vi "Sample Pad Example (LINX).vi"() -> ()   [LabVIEW 2020]
doc: "A simple sample pad, which can trigger up to 16 simultaneous sound effects. Demonstrates the Mixer component, including file loading, playback, and mixer audio monitoring via a music visualizer."
uses:
  Mixer/Channel/Controls/Channel State.ctl
  Mixer/Mixer/Mixer.lvclass/Mixer.ctl
  <vilib>/MakerHub/LINX/Public/Peripherals/Digital/Digital Read N Chans.vi
  e8fa8eb6-c38c-4b8a-b362-922d187964a0.vi
  <vilib>/MakerHub/LINX/Private/Local IO/LinxDigitalRead.vi
  <vilib>/MakerHub/LINX/Public/Utilities/Check Channel.vi
  Mixer/Mixer/Polymorphic VIs/Channel Load (Path).vi
  <vilib>/MakerHub/LINX/Public/Utilities/Open Local.vi
  <vilib>/MakerHub/LINX/Private/Utilties/Generate Error.vi
  Mixer/Mixer/Mixer.lvclass
  Mixer/Channel/Channel.lvclass
  <vilib>/MakerHub/LINX/LMH-LINX.lvlib
panel:
  in  "Sample Path":path=path "/home/pi/samples"
  in  "Stop":bool
  in  "Play 4":bool caption="V"
  in  "Play 3":bool caption="C"
  in  "Play 2":bool caption="X"
  in  "Play 1":bool caption="Z"
  in  "Play 8":bool caption="F"
  in  "Play 7":bool caption="D"
  in  "Play 6":bool caption="S"
  in  "Play 5":bool caption="A"
  in  "Play 12":bool caption="R"
  in  "Play 11":bool caption="E"
  in  "Play 10":bool caption="W"
  in  "Play 9":bool caption="Q"
  in  "Play 16":bool caption="4"
  in  "Play 15":bool caption="3"
  in  "Play 14":bool caption="2"
  in  "Play 13":bool caption="1"
  # "Instructions:\n1. Ensure G-Audio has been installed on the LINX target.\n2. Enter the path to a folder of audio files on the LINX target\n    (e.g. /home/pi/samples).\n3. Run the VI.\n4. Click the buttons below to trigger playback.\n5. (Optional) Wire buttons to the device's DI channels."
  # "G"
  # "-Audio"
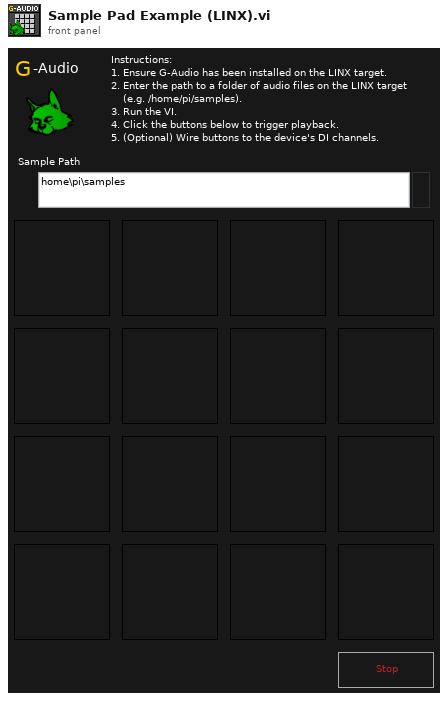
[diagram p1: front panel]
types:
  T1 = typedef "G-Audio.lvlib/Channel.lvclass/Channel State.ctl" = enum16{"Empty", "Error", "Loading", "Loaded", "Stopped", "Paused", "Playing", "Retrigger"}
  T2 = typedef "LMH-LINX.lvlib/LINX Ref.ctl" = cluster{"IO":T3, "Interface":T4, "LINX Device Config":T5}
  T3 = typedef "LMH-LINX.lvlib/Platform.ctl" = enum16{"Remote", "Local"}
  T4 = typedef "LMH-LINX.lvlib/Interface.ctl" = enum16{"Serial", "TCP"}
  T5 = typedef "LMH-LINX.lvlib/Device.lvlib/LINX Device Config.ctl" = cluster{"Interface":T4, "COM Port":refnum<visa-resource-name>, "TCP Configuration":T6, "Device Family":u8, "Device ID":u8, "Device Name":string, "TCP Ref":refnum<k5>, "Channels":T7}
  T6 = typedef "LMH-LINX.lvlib/Device.lvlib/TCP Config.ctl" = cluster{"IP Address":string, "Port":u16}
  T7 = typedef "LMH-LINX.lvlib/Channels.ctl" = cluster{"DI":u8[], "DO":u8[], "AI":u8[], "AO":u8[], "PWM":u8[], "QE":u8[], "UART":u8[], "I2C 2":u8[], "SPI":u8[], "CAN":u8[], "Servo":u8[], "AI Ref (V)":dbl, "AI Resolution (Bits)":u8, "AO Ref (V)":dbl, "AO Resolution (Bits)":u8}
  T8 = typedef "G-Audio.lvlib/Channel.lvclass/Channel Status.ctl" = cluster{"Frame":u64, "State":T1, "Volume":dbl}
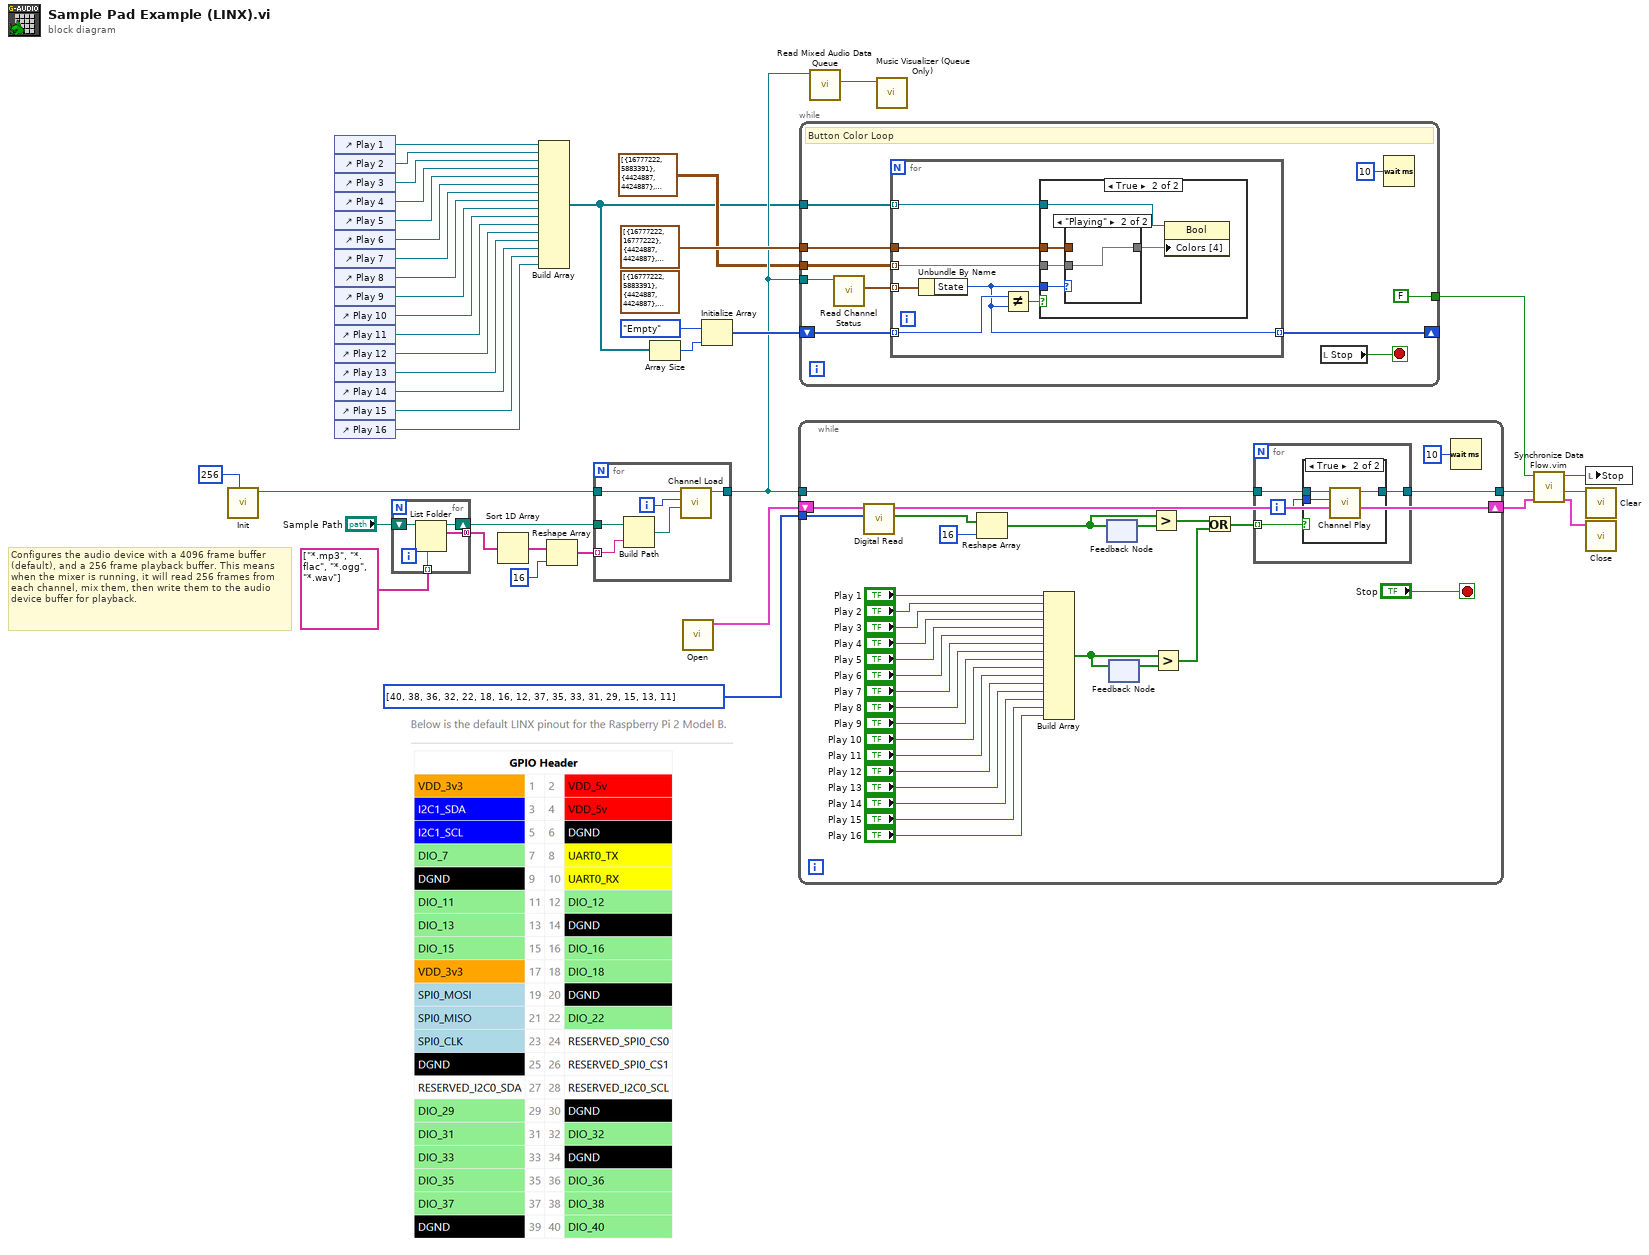
[diagram p0: block diagram]
diagram:
  (unwired) cluster{"Color Box":u32, "Color Box":u32}[][] [[{"Color Box"=16777222, "Color Box"=5883391}, {"Color Box"=4424887, "Color Box"=4424887}, {"Color Box"=4424887, "Color Box"=4424887}, {"Color Box"=4424887, "Color Box"=4424887}], [{"Color Box"=16777222, "Color Box"=5883391}, {"Color Box"=4424887, "Color Box"=4424887}, {"Color Box"=4424887, "Color Box"=4424887}, {"Color Box"=4424887, "Color Box"=4424887}], [{"Color Box"=16777222, "Color Box"=5883391}, {"Color Box"=4424887, "Color Box"=4424887}, {"Color Box"=4424887, "Color Box"=4424887}, {"Color Box"=4424887, "Color Box"=4424887}], [{"Color Box"=16777222, "Color Box"=5883391}, {"Color Box"=4424887, "Color Box"=4424887}, {"Color Box"=4424887, "Color Box"=4424887}, {"Color Box"=4424887, "Color Box"=4424887}], [{"Color Box"=16777222, "Color Box"=6618880}, {"Color Box"=4424887, "Color Box"=4424887}, {"Color Box"=4424887, "Color Box"=4424887}, {"Color Box"=4424887, "Color Box"=4424887}], [{"Color Box"=16777222, "Color Box"=6618880}, {"Color Box"=4424887, "Color Box"=4424887}, {"Color Box"=4424887, "Color Box"=4424887}, {"Color Box"=4424887, "Color Box"=4424887}], [{"Color Box"=16777222, "Color Box"=6618880}, {"Color Box"=4424887, "Color Box"=4424887}, {"Color Box"=4424887, "Color Box"=4424887}, {"Color Box"=4424887, "Color Box"=4424887}], [{"Color Box"=16777222, "Color Box"=6618880}, {"Color Box"=4424887, "Color Box"=4424887}, {"Color Box"=4424887, "Color Box"=4424887}, {"Color Box"=4424887, "Color Box"=4424887}], [{"Color Box"=16777222, "Color Box"=16746514}, {"Color Box"=4424887, "Color Box"=4424887}, {"Color Box"=4424887, "Color Box"=4424887}, {"Color Box"=4424887, "Color Box"=4424887}], [{"Color Box"=16777222, "Color Box"=16746514}, {"Color Box"=4424887, "Color Box"=4424887}, {"Color Box"=4424887, "Color Box"=4424887}, {"Color Box"=4424887, "Color Box"=4424887}], [{"Color Box"=16777222, "Color Box"=16746514}, {"Color Box"=4424887, "Color Box"=4424887}, {"Color Box"=4424887, "Color Box"=4424887}, {"Color Box"=4424887, "Color Box"=4424887}], [{"Color Box"=16777222, "Color Box"=16746514}, {"Color Box"=4424887, "Color Box"=4424887}, {"Color Box"=4424887, "Color Box"=4424887}, {"Color Box"=4424887, "Color Box"=4424887}], [{"Color Box"=16777222, "Color Box"=16711680}, {"Color Box"=4424887, "Color Box"=4424887}, {"Color Box"=4424887, "Color Box"=4424887}, {"Color Box"=4424887, "Color Box"=4424887}], [{"Color Box"=16777222, "Color Box"=16711680}, {"Color Box"=4424887, "Color Box"=4424887}, {"Color Box"=4424887, "Color Box"=4424887}, {"Color Box"=4424887, "Color Box"=4424887}], [{"Color Box"=16777222, "Color Box"=16711680}, {"Color Box"=4424887, "Color Box"=4424887}, {"Color Box"=4424887, "Color Box"=4424887}, {"Color Box"=4424887, "Color Box"=4424887}], [{"Color Box"=16777222, "Color Box"=16711680}, {"Color Box"=4424887, "Color Box"=4424887}, {"Color Box"=4424887, "Color Box"=4424887}, {"Color Box"=4424887, "Color Box"=4424887}]] ("appended array")
  # "Configures the audio device with a 4096 frame buffer (default), and a 256 frame playback buffer. This means when the mixer is running, it will read 256 frames from each channel, mix them, then write them to the audio device buffer for playback."
  n1 = call "Init.vi"("Playback Size (4096)"=256) -> ("Mixer out"=w6:refnum<class "Mixer.lvclass">)  [unwired: 9 in, 1 out]
  n2 = control-ref of="Play 1"() -> (w30:refnum<vi>)
  n3 = control-ref of="Play 2"() -> (w29:refnum<vi>)
  n4 = control-ref of="Play 3"() -> (w28:refnum<vi>)
  n5 = control-ref of="Play 4"() -> (w27:refnum<vi>)
  n6 = control-ref of="Play 5"() -> (w26:refnum<vi>)
  n7 = control-ref of="Play 6"() -> (w25:refnum<vi>)
  n8 = control-ref of="Play 7"() -> (w24:refnum<vi>)
  n9 = control-ref of="Play 8"() -> (w23:refnum<vi>)
  n10 = control-ref of="Play 9"() -> (w22:refnum<vi>)
  n11 = control-ref of="Play 10"() -> (w21:refnum<vi>)
  n12 = control-ref of="Play 11"() -> (w20:refnum<vi>)
  n13 = control-ref of="Play 12"() -> (w19:refnum<vi>)
  n14 = control-ref of="Play 13"() -> (w18:refnum<vi>)
  n15 = control-ref of="Play 14"() -> (w17:refnum<vi>)
  n16 = control-ref of="Play 15"() -> (w16:refnum<vi>)
  n17 = control-ref of="Play 16"() -> (w15:refnum<vi>)
  n18 = for {
    shift-right: [w45] -> w11
    shift-left: "Sample Path" -> [w44]
    tunnel: string[] ["*.mp3", "*.flac", "*.ogg", "*.wav"] -> [w43] mode=indexing
    tunnel: [w42] -> w8 mode=concatenating
    n19 = List Folder(path=w44, pattern=w43) -> (path out=w45:path, filenames=w42:string[])  [unwired: 2 in, 2 out]
  }
  n20 = Sort 1D Array(array=w8) -> (sorted array=w7:string[])
  n21 = Build Array(w30, w29, w28, w27, w26, w25, w24, w23, w22, w21, w20, w19, w18, w17, w16, w15) -> (w1:refnum<vi>[])
  n22 = Reshape Array(w7, 16 ("dimension size")) -> (w12:string[])
  n23 = for {
    tunnel: w12 -> [w51] mode=indexing
    tunnel: w11 -> [w50]
    tunnel: w6 -> [w49]
    tunnel: [w46] -> w4
    i -> [w48]
    n24 = Build Path(base path=w50, name or relative path=w51) -> (appended path=w47:path)
    n25 = call-poly "Channel Load.vi"("Path"=w47, "Channel Index"=w48, "Mixer in"=w49) -> ("Mixer out"=w46:refnum<class "Mixer.lvclass">)  [unwired: 7 in, 1 out]
  }
  n26 = Array Size(array=w1) -> (size(s)=w36:i32)
  n27 = call-poly <vilib>:"Open.vi"() -> ("LINX Resource"=w31:T2)  [unwired: 9 in, 2 out]
  n28 = Initialize Array(Channel_State."Empty" ("State"), w36) -> (w41:T1[])
  n29 = while {
    tunnel: u8[] [40, 38, 36, 32, 22, 18, 16, 12, 37, 35, 33, 31, 29, 15, 13, 11] -> [w82]
    shift-right: [w80] -> w35
    shift-left: w31 -> [w83]
    tunnel: [w57] -> w33
    tunnel: w4 -> [w56]
    stop <- "Stop" stop-if-true
    n30 = call-poly <vilib>:"Digital Read.vi"("DI Channels"=w82, "LINX Resource"=w83) -> ("Values"=w52:bool[], "LINX Resource"=w80:T2)  [unwired: 7 in, 1 out]
    n31 = Reshape Array(w52, 16 ("dimension size")) -> (w54:bool[])
    n32 = Build Array("Play 1", "Play 2", "Play 3", "Play 4", "Play 5", "Play 6", "Play 7", "Play 8", "Play 9", "Play 10", "Play 11", "Play 12", "Play 13", "Play 14", "Play 15", "Play 16") -> (w61:bool[])
    n33 = feedback-in #1(w54) -> ()
    n34 = feedback #1() -> (w81:bool[])  [unwired: 1 in]
    n35 = feedback #2() -> (w62:bool[])  [unwired: 1 in]
    n36 = feedback-in #2(w61) -> ()
    n37 = Greater?(x=w54, y=w81) -> (0:w60:bool[])
    n38 = Greater?(x=w61, y=w62) -> (0:w59:bool[])
    n39 = Or(x=w60, y=w59) -> (x .or. y?=w58:bool[])
    n40 = for {
      tunnel: w58 -> [w87] mode=indexing
      tunnel: [w85] -> w57
      tunnel: w56 -> [w84]
      i -> [w86]
      n41 = case shown="True" w87 {
        tunnel: w86 -> [_ w91]
        tunnel: [w88 w90] -> w85
        tunnel: w84 -> [w88 w89]
        frame False {
        }
        frame True {
          n42 = call "Channel Play.vi"("Channel Index"=w91, "Mixer in"=w89) -> ("Mixer out"=w90:refnum<class "Mixer.lvclass">)  [unwired: 8 in, 1 out]
        }
      }
    }
    n43 = Wait (ms)(milliseconds to wait=u32 10) -> ()  [unwired: 1 out]
  }
  n44 = while {
    tunnel: w4 -> [w101]
    tunnel: w1 -> [w99]
    tunnel: cluster{u32, u32}[] [{16777222, 16777222}, {4424887, 4424887}, {4424887, 4424887}, {4424887, 4424887}] ("Colors [4]") -> [w98]
    tunnel: cluster{"Color Box":u32, "Color Box":u32}[][] [[{"Color Box"=16777222, "Color Box"=5883391}, {"Color Box"=4424887, "Color Box"=4424887}, {"Color Box"=4424887, "Color Box"=4424887}, {"Color Box"=4424887, "Color Box"=4424887}], [{"Color Box"=16777222, "Color Box"=6618880}, {"Color Box"=4424887, "Color Box"=4424887}, {"Color Box"=4424887, "Color Box"=4424887}, {"Color Box"=4424887, "Color Box"=4424887}], [{"Color Box"=16777222, "Color Box"=16746514}, {"Color Box"=4424887, "Color Box"=4424887}, {"Color Box"=4424887, "Color Box"=4424887}, {"Color Box"=4424887, "Color Box"=4424887}], [{"Color Box"=16777222, "Color Box"=16722505}, {"Color Box"=4424887, "Color Box"=4424887}, {"Color Box"=4424887, "Color Box"=4424887}, {"Color Box"=4424887, "Color Box"=4424887}], [{"Color Box"=16777222, "Color Box"=5883391}, {"Color Box"=4424887, "Color Box"=4424887}, {"Color Box"=4424887, "Color Box"=4424887}, {"Color Box"=4424887, "Color Box"=4424887}], [{"Color Box"=16777222, "Color Box"=6618880}, {"Color Box"=4424887, "Color Box"=4424887}, {"Color Box"=4424887, "Color Box"=4424887}, {"Color Box"=4424887, "Color Box"=4424887}], [{"Color Box"=16777222, "Color Box"=16746514}, {"Color Box"=4424887, "Color Box"=4424887}, {"Color Box"=4424887, "Color Box"=4424887}, {"Color Box"=4424887, "Color Box"=4424887}], [{"Color Box"=16777222, "Color Box"=16722505}, {"Color Box"=4424887, "Color Box"=4424887}, {"Color Box"=4424887, "Color Box"=4424887}, {"Color Box"=4424887, "Color Box"=4424887}], [{"Color Box"=16777222, "Color Box"=5883391}, {"Color Box"=4424887, "Color Box"=4424887}, {"Color Box"=4424887, "Color Box"=4424887}, {"Color Box"=4424887, "Color Box"=4424887}], [{"Color Box"=16777222, "Color Box"=6618880}, {"Color Box"=4424887, "Color Box"=4424887}, {"Color Box"=4424887, "Color Box"=4424887}, {"Color Box"=4424887, "Color Box"=4424887}], [{"Color Box"=16777222, "Color Box"=16746514}, {"Color Box"=4424887, "Color Box"=4424887}, {"Color Box"=4424887, "Color Box"=4424887}, {"Color Box"=4424887, "Color Box"=4424887}], [{"Color Box"=16777222, "Color Box"=16722505}, {"Color Box"=4424887, "Color Box"=4424887}, {"Color Box"=4424887, "Color Box"=4424887}, {"Color Box"=4424887, "Color Box"=4424887}], [{"Color Box"=16777222, "Color Box"=5883391}, {"Color Box"=4424887, "Color Box"=4424887}, {"Color Box"=4424887, "Color Box"=4424887}, {"Color Box"=4424887, "Color Box"=4424887}], [{"Color Box"=16777222, "Color Box"=6618880}, {"Color Box"=4424887, "Color Box"=4424887}, {"Color Box"=4424887, "Color Box"=4424887}, {"Color Box"=4424887, "Color Box"=4424887}], [{"Color Box"=16777222, "Color Box"=16746514}, {"Color Box"=4424887, "Color Box"=4424887}, {"Color Box"=4424887, "Color Box"=4424887}, {"Color Box"=4424887, "Color Box"=4424887}], [{"Color Box"=16777222, "Color Box"=16722505}, {"Color Box"=4424887, "Color Box"=4424887}, {"Color Box"=4424887, "Color Box"=4424887}, {"Color Box"=4424887, "Color Box"=4424887}]] ("appended array") -> [w97]
    tunnel: [FALSE ("Stop")] -> w38
    shift-right: [w93] -> _
    shift-left: w41 -> [w92]
    stop <- w95 stop-if-true
    # "Button Color Loop"
    n45 = call "Read Channel Status.vi"("Mixer in"=w101) -> ("Channel Status"=w100:T8[])  [unwired: 8 in, 2 out]
    n46 = for {
      tunnel: w100 -> [w108] mode=indexing
      tunnel: w99 -> [w107] mode=indexing
      tunnel: w98 -> [w106]
      tunnel: w97 -> [w105] mode=indexing
      tunnel: [w102] -> w93 mode=indexing
      tunnel: w92 -> [w104] mode=indexing
      n47 = Unbundle By Name(w108) -> ("State"=w102:T1)
      n48 = Not Equal?(x=w104, y=w102) -> (x != y?=w103:bool)
      n49 = case shown="True" w103 {
        tunnel: w107 -> [_ w113]
        tunnel: w106 -> [_ w112]
        tunnel: w105 -> [_ w110]
        tunnel: w102 -> [_ w109]
        frame False {
        }
        frame True {
          n50 = case shown="\"Playing\"" w109 {
            tunnel: w112 -> [w114 _]
            tunnel: [w114 w115] -> w111
            tunnel: w110 -> [_ w115]
            frame Default {
            }
            frame "Playing" {
            }
          }
          n51 = property class="Bool"(reference=w113, "Colors [4]"=w111) -> ()  [unwired: 1 in, 2 out]
        }
      }
    }
    n52 = local read "Stop"() -> (w95:bool)
    n53 = Wait (ms)(milliseconds to wait=u32 10) -> ()  [unwired: 1 out]
  }
  n54 = call "Read Mixed Audio Data Queue.vi"("Mixer in"=w4) -> ("Mixed Audio Data"=w3:refnum<queue>)  [unwired: 8 in, 2 out]
  n55 = call "Music Visualizer (Queue Only).vi"("Mixed Audio Data"=w3) -> ()  [unwired: 11 in]
  n56 = call "Synchronize Data Flow.vim"("input 4"=w35, "input 3"=w33, "input 1"=w38) -> ("output 4"=w34:T2, "output 3"=w32:refnum<class "Mixer.lvclass">, "output 1"=w39:bool)  [unwired: 1 in, 1 out]
  n57 = local write "Stop"(w39) -> ()
  n58 = call "Clear.vi"("Mixer in"=w32) -> ()  [unwired: 10 in, 1 out]
  n59 = call <vilib>:"Close.vi"("LINX Resource"=w34) -> ()  [unwired: 10 in, 1 out]
